vi "createIntProperty.vi"(6 "Visible (T)":bool=TRUE, 8 "error in (no error)":errorcluster, 9 "DefaultValue":i64, 10 "Name":string, 11 "IProperty in":refnum<class "IProperty.lvclass">) -> (0 "error out":errorcluster, 3 "IProperty out":refnum<class "IProperty.lvclass">)   [LabVIEW 2022 SP3, in "openDAQ.lvlib" / "IBaseObject.lvlib" / "IProperty.lvlib" / "IProperty.lvclass"]
uses:
  <instrlib>/openDAQ/Public/Classes/IProperty/IProperty.lvclass
  <instrlib>/openDAQ/Public/Classes/IProperty/IProperty.lvclass/IProperty.ctl
  <instrlib>/openDAQ/Public/Classes/daqCoreTypes/IString/IString.lvclass
  <instrlib>/openDAQ/Public/Classes/daqCoreTypes/IBoolean/IBoolean.lvclass
  <instrlib>/openDAQ/Public/Classes/daqCoreTypes/IInteger/IInteger.lvclass
  <instrlib>/openDAQ/Binaries/Windows/x86/copendaq32.dll
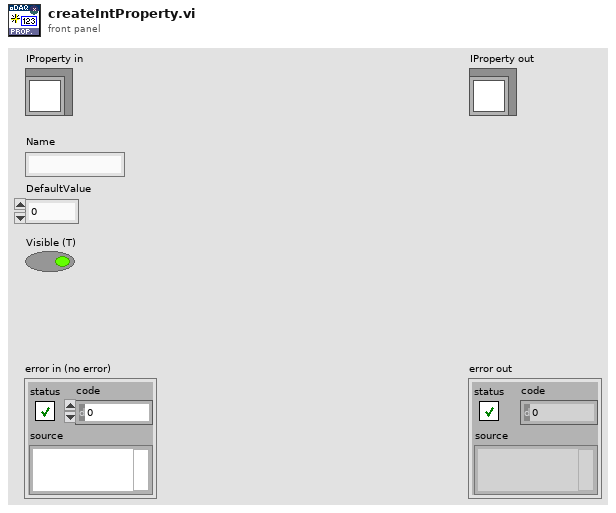
[diagram p1: front panel]
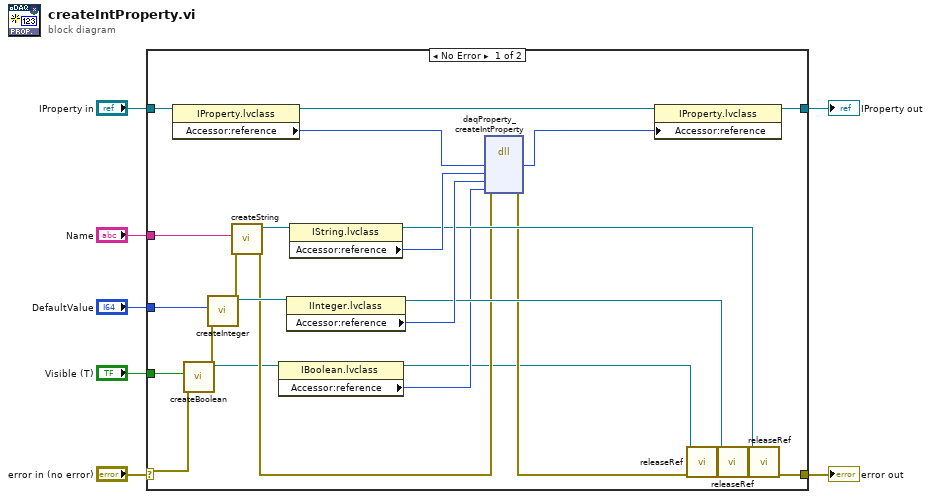
[diagram p0: block diagram]
diagram:
  n1 = case shown="No Error" "error in (no error)" {
    selector: "error in (no error)" -> [w16 w34]
    tunnel: [w19 w34] -> w6
    tunnel: [w30 w33] -> w4
    tunnel: "IProperty in" -> [w32 w33]
    tunnel: "Name" -> [w26 _]
    tunnel: "DefaultValue" -> [w25 _]
    tunnel: "Visible (T)" -> [w14 _]
    frame No Error {
      n2 = property class="IProperty.lvclass"(reference=w32) -> (reference out=w31:refnum<class "IProperty.lvclass">, "Accessor:reference"=w29:i64)  [unwired: 1 in, 1 out]
      n3 = call <instrlib>:"createBoolean.vi"("error in (no error)"=w16, "bool"=w14) -> ("error out"=w15:errorcluster, "IBoolean out"=w12:refnum<class "IBoolean.lvclass">)  [unwired: 8 in]
      n4 = call <instrlib>:"createInteger.vi"("error in (no error)"=w15, "Value"=w25) -> ("error out"=w27:errorcluster, "IInteger out"=w23:refnum<class "IInteger.lvclass">)  [unwired: 8 in]
      n5 = call <instrlib>:"createString.vi"("error in (no error)"=w27, "String"=w26) -> ("error out"=w13:errorcluster, "IString out"=w24:refnum<class "IString.lvclass">)  [unwired: 8 in]
      n6 = property class="IBoolean.lvclass"(reference=w12) -> (reference out=w8:refnum<class "IBoolean.lvclass">, "Accessor:reference"=w11:i64)  [unwired: 1 in, 1 out]
      n7 = property class="IInteger.lvclass"(reference=w23) -> (reference out=w18:refnum<class "IInteger.lvclass">, "Accessor:reference"=w21:i64)  [unwired: 1 in, 1 out]
      n8 = property class="IString.lvclass"(reference=w24) -> (reference out=w17:refnum<class "IString.lvclass">, "Accessor:reference"=w22:i64)  [unwired: 1 in, 1 out]
      n9 = dll-call lib="C:/Program Files (x86)/National Instruments/LabVIEW 2022/instr.lib/openDAQ/Binaries/Windows/x86/copendaq*.*" fn="daqProperty_createIntProperty"(error in=w13, "property"=w29, "propertyName"=w22, "propertyDefaultValue"=w21, "PropertyVisible"=w11) -> (error out=w9:errorcluster, "property"=w28:i64)  [unwired: 6 in, 1 out]
      n10 = property class="IProperty.lvclass"(reference=w31, "Accessor:reference"=w28) -> (reference out=w30:refnum<class "IProperty.lvclass">)  [unwired: 1 in, 1 out]
      n11 = call-dynamic "releaseRef.vi"("error in (no error)"=w9, "IBaseObject in"=w8) -> ("error out"=w10:errorcluster)  [unwired: 9 in]
      n12 = call-dynamic "releaseRef.vi"("error in (no error)"=w10, "IBaseObject in"=w18) -> ("error out"=w20:errorcluster)  [unwired: 9 in]
      n13 = call-dynamic "releaseRef.vi"("error in (no error)"=w20, "IBaseObject in"=w17) -> ("error out"=w19:errorcluster)  [unwired: 9 in]
    }
    frame Error {
    }
  }
  "error out" <- w6
  "IProperty out" <- w4
